vi "TA_Read_Data.vi"(11 "File Path":path=path "\\\\Mac\\Home/Desktop/fs-TA/Data/demo_fsta.dat") -> (3 "TA Data":T1)   [LabVIEW 2025]
uses:
  TA_DATA.ctl
  <vilib>/Utility/file.llb/Read Delimited Spreadsheet (DBL).vi
panel:
  out "Application Directory":path
  out "path":path
  out "size (raw data)":i32[](array[numeric])
  out "raw data":dbl[][](array[numeric]) format="%#_8g"
  in  "delimiter (\\t tab; , comma)":string="\t"
  in  "transpose? (F)":bool
  in  "max characters/row  (no limit:0)":i32
  in  "start of read offset (chars.:0)":i32
  in  "number of rows (all:-1)":i32=-1
  in  "format (%.10f)":string="%.10f"
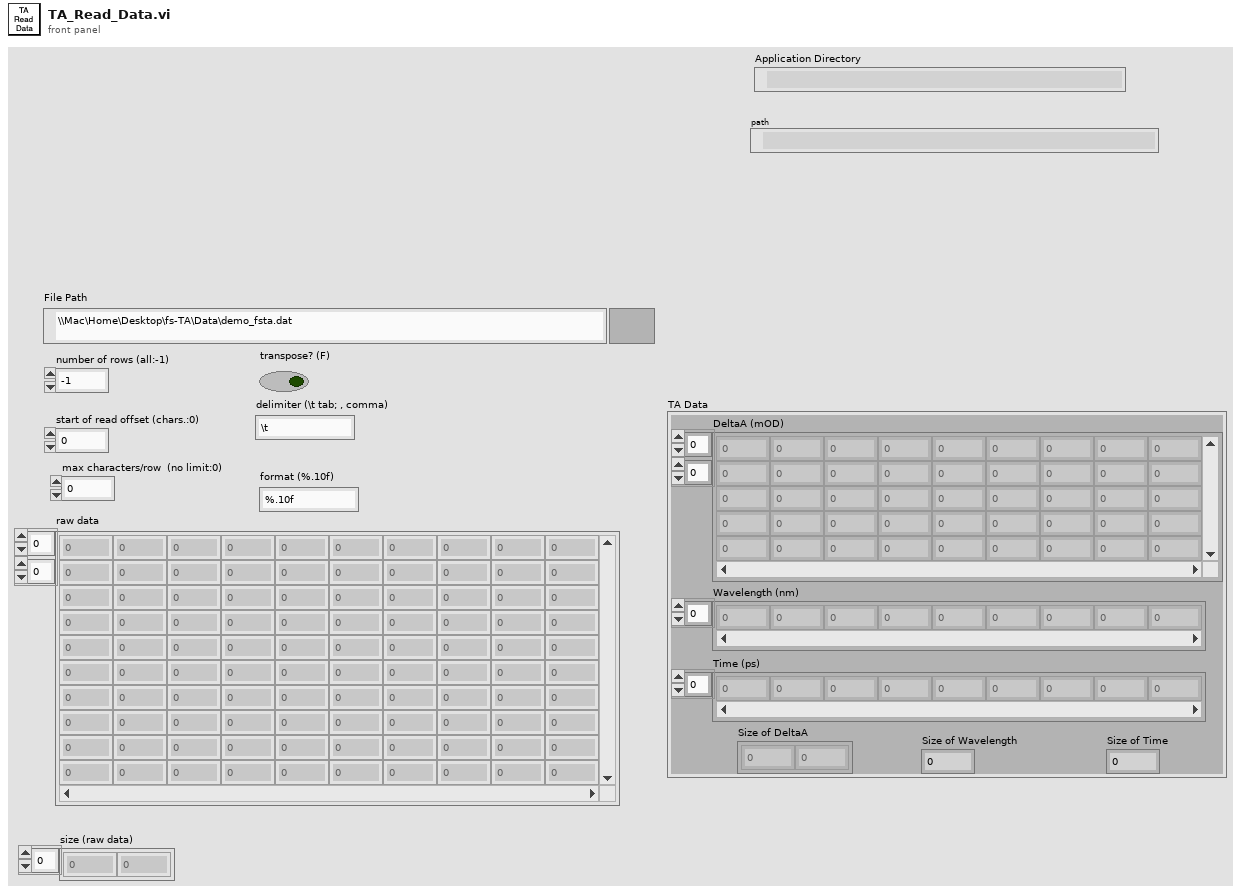
[diagram p1: front panel]
types:
  T1 = typedef "TA_DATA.ctl" = cluster{"DeltaA (mOD)":dbl[][], "Wavelength (nm)":dbl[], "Time (ps)":dbl[], "Size of DeltaA":i32[], "Size of Wavelength":i32, "Size of Time":i32}
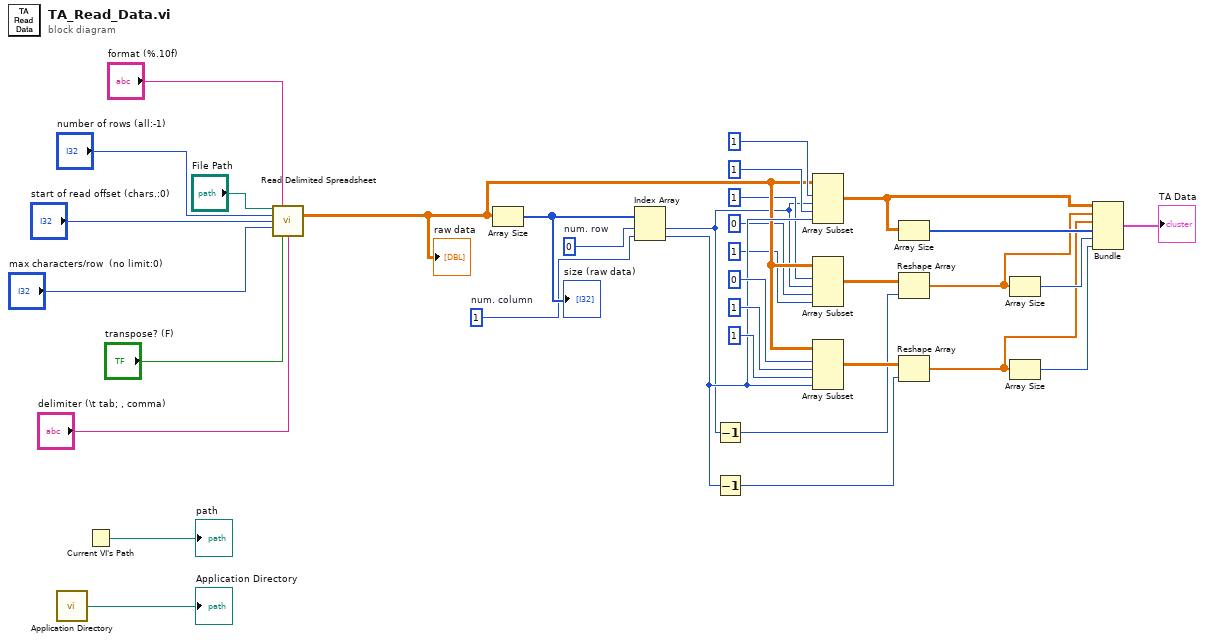
[diagram p0: block diagram]
diagram:
  w20 = 1  # num. column
  w27 = 0  # num. row
  n1 = call <vilib>:"Application Directory.vi"() -> ("Application Directory"=→"Application Directory":path)
  n2 = Current VI's Path() -> (path=→"path":path)
  n3 = call-poly <vilib>:"Read Delimited Spreadsheet.vi"("file path (dialog if empty)"="File Path", "format (%.3f)"="format (%.10f)", "number of rows (all:-1)"="number of rows (all:-1)", "start of read offset (chars.:0)"="start of read offset (chars.:0)", "max characters/row  (no limit:0)"="max characters/row  (no limit:0)", "transpose? (F)"="transpose? (F)", "delimiter (\\t)"="delimiter (\\t tab; , comma)") -> ("all rows"=w14:dbl[][])  [unwired: 3 in, 5 out]
  "raw data" <- w14
  n4 = Array Size(array=w14) -> (size(s)=w24:i32[])
  "size (raw data)" <- w24
  n5 = Index Array "Index Array"(array=w24, index #1=w27, index #2=w20) -> (element #1=w10:i32, element #2=w18:i32)
  n6 = Decrement(x=w10) -> (x-1=w16:i32)
  n7 = Decrement(x=w18) -> (x-1=w17:i32)
  n8 = Array Subset "Array Subset"(array=w14, index (row)=1 ("index"), length (row)=w10, index (col)=1 ("index"), length (col)=w18) -> (w6:dbl[][])
  n9 = Array Subset "Array Subset"(array=w14, index (row)=1 ("index"), length (row)=w10, index (col)=0 ("index"), length (col)=1 ("length")) -> (w15:dbl[][])
  n10 = Array Subset "Array Subset"(array=w14, index (row)=0 ("index"), length (row)=1 ("length"), index (col)=1 ("index"), length (col)=w18) -> (w23:dbl[][])
  n11 = Array Size(array=w6) -> (size(s)=w9:i32[])
  n12 = Reshape Array "Reshape Array"(w15, w16) -> (w5:dbl[])
  n13 = Reshape Array "Reshape Array"(w23, w17) -> (w4:dbl[])
  n14 = Array Size(array=w5) -> (size(s)=w8:i32)
  n15 = Array Size(array=w4) -> (size(s)=w7:i32)
  n16 = Bundle(w6, w5, w4, w9, w8, w7) -> (→"TA Data":cluster{dbl[][], dbl[], dbl[], i32[], i32, i32})  [unwired: 1 in]
